vi "Validate Plate Tank Enable.vi"(8 "Valve No.":i32, 9 "Test Value":bool, 10 "Tag":string, 11 "Queue in":T1) -> ()   [LabVIEW 2019]
uses:
  <vilib>/NI/AMC/Message Queue.ctl
  <vilib>/NI/AMC/Message.ctl
  <vilib>/NI/Tools/Keyed Array/KeyedArray.ctl
  <vilib>/NI/Tools/Keyed Array/Tools_KeyedArray.lvlib
  <vilib>/NI/AMC/AMC.lvlib
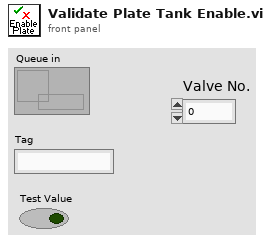
[diagram p1: front panel]
types:
  T1 = typedef "AMC.lvlib/Message Queue.ctl" = refnum<queue>
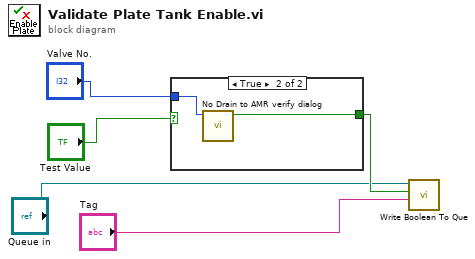
[diagram p0: block diagram]
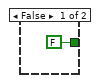
[diagram p2: hidden frame]
diagram:
  n1 = case shown="True" "Test Value" {
    tunnel: [FALSE ("Drain?") w8] -> w4
    tunnel: "Valve No." -> [_ w7]
    frame False {
    }
    frame True {
      n2 = call "No Drain to AMR verify dialog.vi"("d"=w7) -> ("Drain?"=w8:bool)  [unwired: 10 in]
    }
  }
  n3 = call "Write Boolean To Que.vi"("Tag"="Tag", "NewVal"=w4, "Queue in"="Queue in") -> ()  [unwired: 9 in]
